vi "seletor_de_sinais.vi"() -> ()   [LabVIEW 2025]
panel:
  in  "stop":bool
  in  "Phase":dbl
  in  "Offset":dbl
  in  "Frequency":dbl format="%#_13g"
  in  "Amplitude":dbl
  in  "Enum":T1(ring)
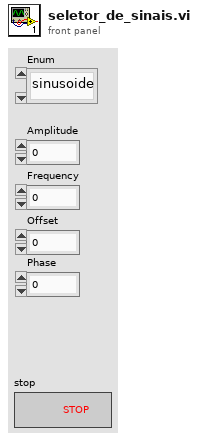
[diagram p1: front panel]
types:
  T1 = enum16{"sinusoide", "quadrada", "triangular", "sawtooth"}
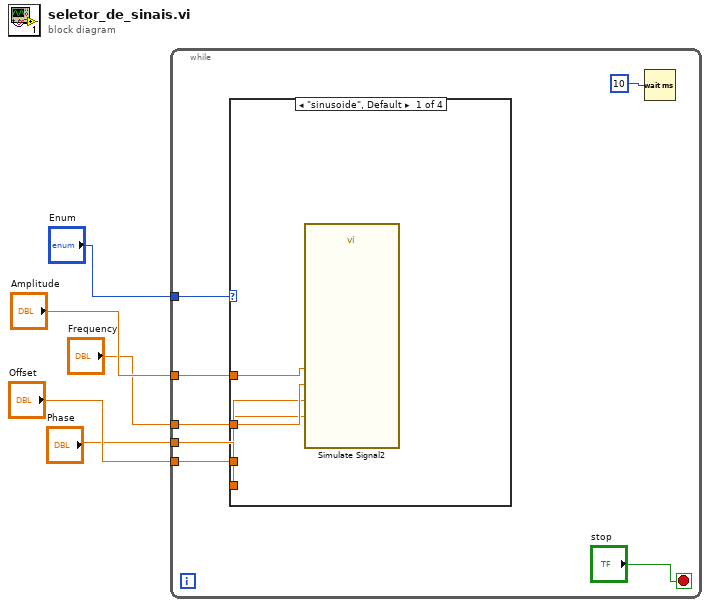
[diagram p0: block diagram]
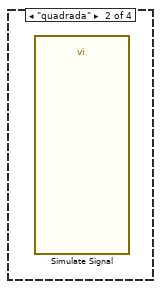
[diagram p2: hidden frame]
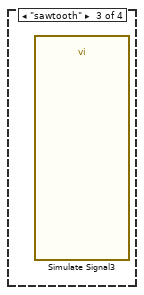
[diagram p3: hidden frame]
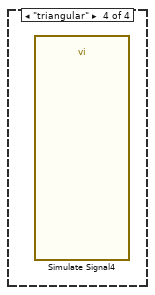
[diagram p4: hidden frame]
diagram:
  n1 = while {
    tunnel: "Enum" -> [w12]
    tunnel: "Amplitude" -> [w11]
    tunnel: "Frequency" -> [w10]
    tunnel: "Offset" -> [w9]
    tunnel: "Phase" -> [w8]
    stop <- "stop" stop-if-true
    n2 = case shown="\"sinusoide\", Default" w12 {
      tunnel: w11 -> [w16 _ _ _]
      tunnel: w10 -> [w15 _ _ _]
      tunnel: w9 -> [w14 _ _ _]
      tunnel: w8 -> [w13 _ _ _]
      frame "sinusoide", Default {
        n3 = call "Simulate Signal2"("Offset"=w14, "Frequency"=w15, "Amplitude"=w16, "Phase"=w13) -> ()  [unwired: 10 in, 2 out]
      }
      frame "quadrada" {
        n4 = call "Simulate Signal"() -> ()  [unwired: 14 in, 2 out]
      }
      frame "sawtooth" {
        n5 = call "Simulate Signal3"() -> ()  [unwired: 14 in, 2 out]
      }
      frame "triangular" {
        n6 = call "Simulate Signal4"() -> ()  [unwired: 14 in, 2 out]
      }
    }
    n7 = Wait (ms)(milliseconds to wait=u32 10) -> ()  [unwired: 1 out]
  }
